vi "Add Caption and image.vi"(0 "PDF Report IN":T21(xcontrol), 2 "Caption?":bool, 5 "Paragraph Refnum":refnum<k24>, 9 "Image Ref iTexSharp":refnum<k24>, 11 "error in (no error)":errorcluster) -> (4 "PDF Report OUT":T21(xcontrol), 8 "Size (points)":cluster{"TotalHeight":sgl, "TotalWidth":sgl}, 15 "error out":errorcluster)   [LabVIEW 2012]
doc: "Version 1.0\nDeveloped by Jean-Marc Simard\nCopyright © 2010, Exaprom Inc.\nAll rights reserved.\nLicense: BSD\n\nWith iTextSharp 4.1.6 (http://itextsharp.sourceforge.net)\nunder Mozilla Public License Version 1.1\n(http://www.mozilla.org/MPL/MPL-1.1.html)"
uses:
  C:/Users/MaxCorp/Documents/GitHub/TopView/DLL/itextsharp.dll
  GitHub/TopView/DLL/itextsharp.dll
  Controls/PDF Report Xcontrol/PDF Report.xctl
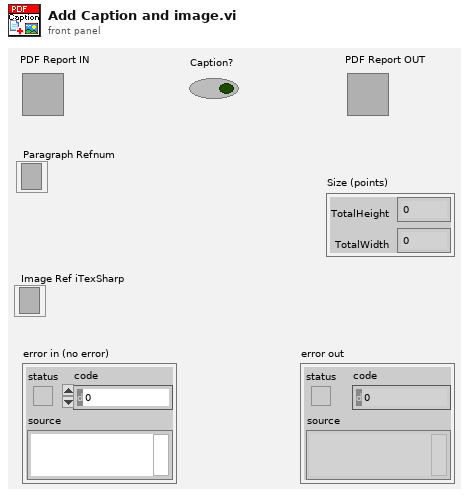
[diagram p1: front panel]
types:
  T1 = typedef "Font cluster.ctl" = cluster{"Name":string, "Size":T2, "Color":T3, "Style":cluster{"Bold":bool, "Italic":bool, "Underline":bool, "Strikeout":bool}}
  T2 = typedef "Font size.ctl" = sgl
  T3 = typedef "Font color.ctl" = u32
  T4 = typedef "Unit.ctl" = enum16{"inch", "mm"}
  T5 = typedef "Paragraphe cluster.ctl" = cluster{" Aligment":T6, "Line spacing":T7}
  T6 = typedef "Texte alignement.ctl" = enum16{"Select", "CENTER", "JUSTIFY", "LEFT", "RIGHT"}
  T7 = typedef "Line spacing.ctl" = enum16{"Select", "1.0", "1.5", "2.0"}
  T8 = typedef "Page dimensions.ctl" = cluster{"Start at page":i32, "Orientation":T9, "widht":sgl, "height":sgl, "Margin left":sgl, "Margin right":sgl, "Margin top":sgl, "Margin bottom":sgl}
  T9 = typedef "Page Orientation.ctl" = enum16{"Portrait", "Landscape"}
  T10 = typedef "Image or Table Caption.ctl" = cluster{"Caption":string, "Separator":string, "Position":enum16{"Above", "Below"}}
  T11 = typedef "Header Footer [ ].ctl" = T12[]
  T12 = typedef "Header Footer cluster.ctl" = cluster{"Start page":i32, "Type":T13, "Alignment":T14, "Vertical Alignement":T15, "Image (%)":sgl, "Page #":T16, "Text":string, "Path":string, "Font":T1, "Font refnum":refnum<k24>, "Line":cluster{"Line":T17, "Thickness (points)":sgl, "Colour":T3}}
  T13 = typedef "Header Footer Type.ctl" = enum16{"Select", "Text", "Text + hyperlink", "Page number", "Image", "Image + hyperlink"}
  T14 = typedef "Header footer horiz alignment.ctl" = enum16{"Left", "Center", "Right"}
  T15 = typedef "Cell Vertical alignment.ctl" = enum16{"TOP", "MIDDLE", "BOTTOM"}
  T16 = typedef "Page number.ctl" = cluster{"Text 1":string, "Text 2":string, "Text 3":string}
  T17 = typedef "Header Footer Line.ctl" = enum16{"No line", "Horizontal line"}
  T18 = typedef "Watermark cluster2.ctl" = cluster{"Show? (F)":bool, "Type":enum16{"Image", "Text"}, "Opacity (%)":sgl, "Rotate(°)":sgl, "Position":cluster{"Position":T19, "X":sgl, "Y":sgl}, "Image path":path, "Scaled(%)":sgl, "Image refnum":refnum<k24>, "Text":string, "Font":cluster{"Name":string, "Size":T2, "Color":T3}, "Font refnum":refnum<k24>, "Alignment":T14, "Automatic":bool}
  T19 = typedef "Watermark Position.ctl" = enum16{"Absolute", "Center (page)", "Center (text section)"}
  T20 = typedef "System Fonts.ctl" = cluster{"Font name [ ]":string[], "Font and file names [ ]":cluster{"Font name":string, "File name":string}[]}
  T21 = cluster{"Document":refnum<k24>, "Writer":refnum<k24>, "Default Font":refnum<k24>, "Default Font cluster":T1, "Path":path, "Unit (default = mm)":T4, "Paragraphe cluster":T5, "Pages dimensions [ ]":T8[], "Captions":cluster{"Image":T10, "Image counter":u16, "Table":T10, "Table counter":u16, "Font":T1}, "Header":T11, "Footer":T11, "Watermark ":T18, "Actual VI name":string, "System Fonts":T20}
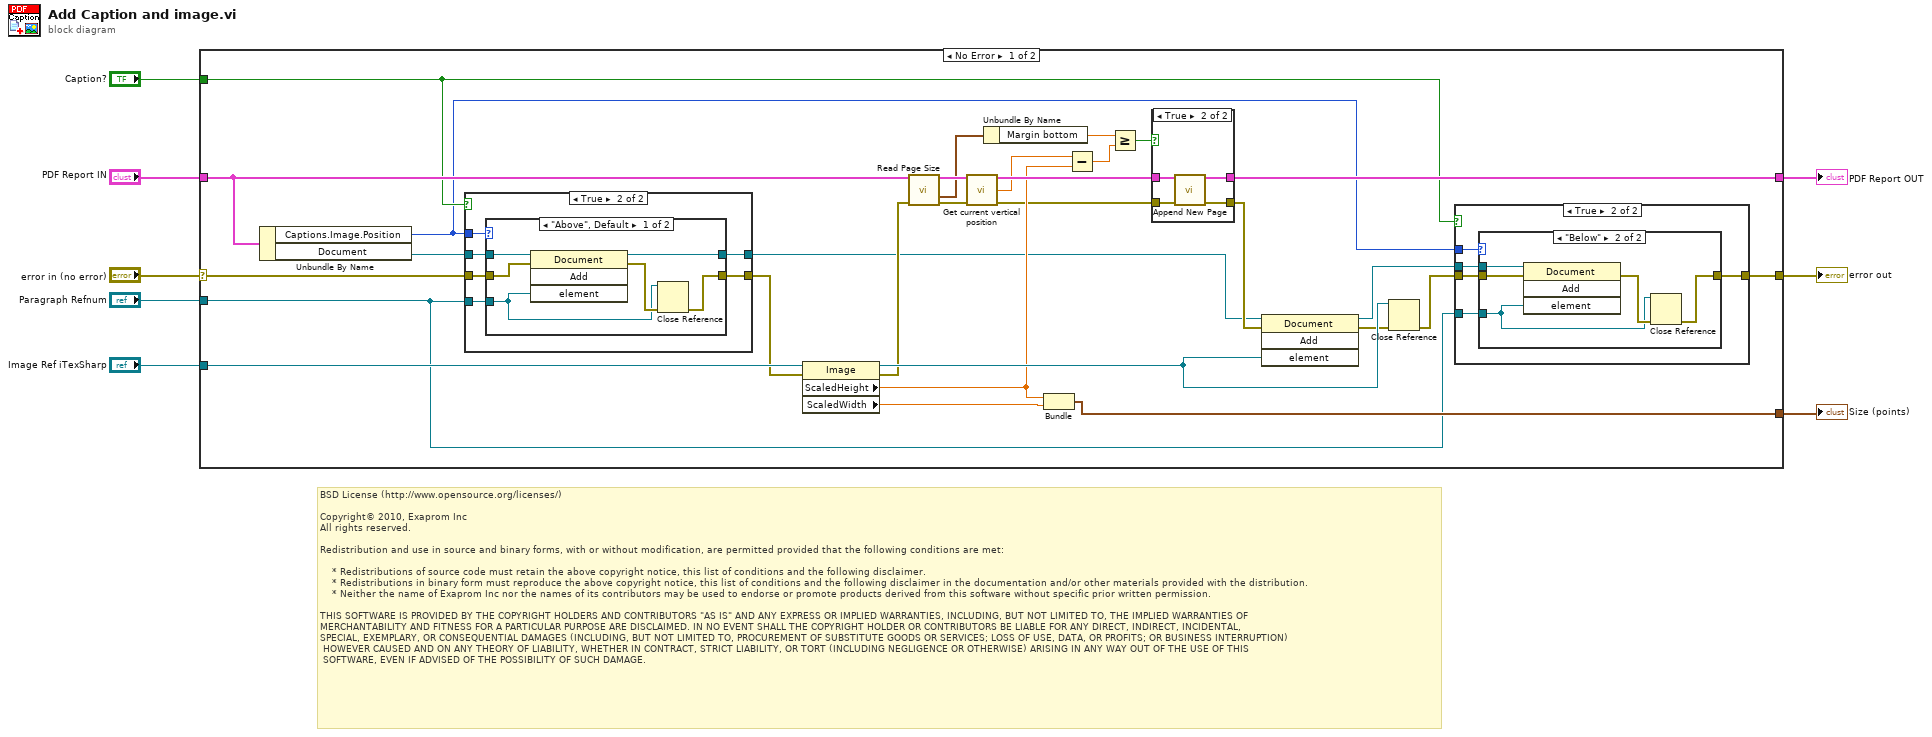
[diagram p0: block diagram]
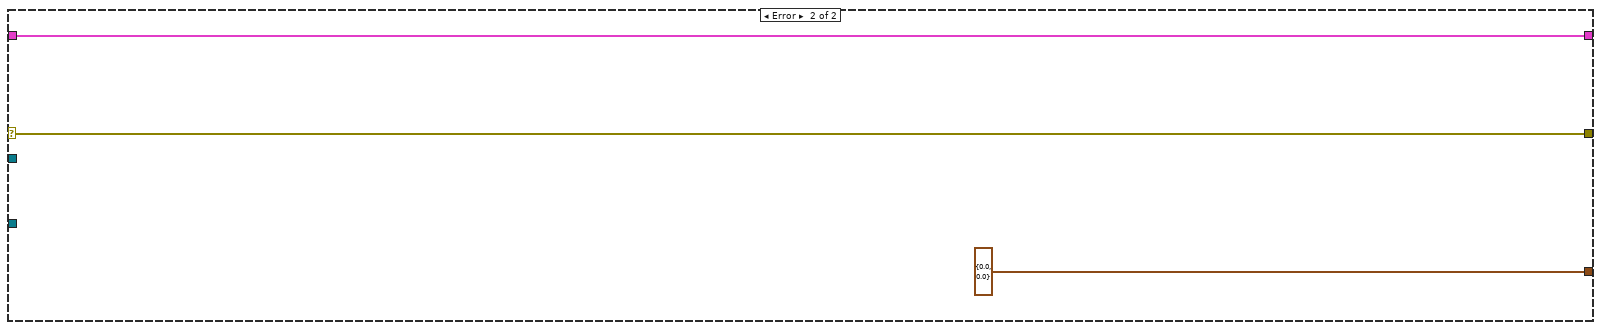
[diagram p7: hidden frame]
diagram:
  # "BSD License (http://www.opensource.org/licenses/)\n\nCopyright© 2010, Exaprom Inc\nAll rights reserved.\n\nRedistribution and use in source and binary forms, with or without modification, are permitted provided that the following conditions are met:\n\n    * Redistributions of source code must retain the above copyright notice, this list of conditions and the following disclaimer.\n    * Redistributions in binary form must reproduce the above copyright notice, this list of conditions and the following disclaimer in the documentation and/or other materials provided with the distribution.\n    * Neither the name of Exaprom Inc nor the names of its contributors may be used to endorse or promote products derived from this software without specific prior written permission.\n\nTHIS SOFTWARE IS PROVIDED BY THE COPYRIGHT HOLDERS AND CONTRIBUTORS \"AS IS\" AND ANY EXPRESS OR IMPLIED WARRANTIES, INCLUDING, BUT NOT LIMITED TO, THE IMPLIED WARRANTIES OF \nMERCHANTABILITY AND FITNESS FOR A PARTICULAR PURPOSE ARE DISCLAIMED. IN NO EVENT SHALL THE COPYRIGHT HOLDER OR CONTRIBUTORS BE LIABLE FOR ANY DIRECT, INDIRECT, INCIDENTAL,\nSPECIAL, EXEMPLARY, OR CONSEQUENTIAL DAMAGES (INCLUDING, BUT NOT LIMITED TO, PROCUREMENT OF SUBSTITUTE GOODS OR SERVICES; LOSS OF USE, DATA, OR PROFITS; OR BUSINESS INTERRUPTION)\n HOWEVER CAUSED AND ON ANY THEORY OF LIABILITY, WHETHER IN CONTRACT, STRICT LIABILITY, OR TORT (INCLUDING NEGLIGENCE OR OTHERWISE) ARISING IN ANY WAY OUT OF THE USE OF THIS\n SOFTWARE, EVEN IF ADVISED OF THE POSSIBILITY OF SUCH DAMAGE."
  n1 = case shown="No Error" "error in (no error)" {
    selector: "error in (no error)" -> [w31 w74]
    tunnel: "PDF Report IN" -> [w34 w73]
    tunnel: [w37 w73] -> w7
    tunnel: [w35 w74] -> w6
    tunnel: [w36 cluster{"ScaledHeight":sgl, "ScaledWidth":sgl} {"ScaledHeight"=0.0, "ScaledWidth"=0.0}] -> w3
    tunnel: "Image Ref iTexSharp" -> [w32 _]
    tunnel: "Caption?" -> [w29 _]
    tunnel: "Paragraph Refnum" -> [w30 _]
    frame No Error {
      n2 = Unbundle By Name(w34) -> ("Captions.Image.Position"=w9:enum16{"Above", "Below"}, "Document"=w33:refnum<k24>)
      n3 = case shown="True" w29 {
        tunnel: w31 -> [w50 w57]
        tunnel: w33 -> [w51 w56]
        tunnel: [w50 w55] -> w13
        tunnel: [w51 w54] -> w12
        tunnel: w9 -> [_ w53]
        tunnel: w30 -> [_ w52]
        frame False {
        }
        frame True {
          n4 = case shown="\"Above\", Default" w53 {
            tunnel: w52 -> [w62 _]
            tunnel: w57 -> [w61 w64]
            tunnel: [w60 w64] -> w55
            tunnel: w56 -> [w59 w65]
            tunnel: [w58 w65] -> w54
            frame "Above", Default {
              n5 = invoke class="Document" method="Add"(reference=w59, error in=w61, "element"=w62) -> (reference out=w58:refnum<k24>, error out=w63:errorcluster)  [unwired: 1 in, 2 out]
              n6 = Close Reference(reference=w62, error in (no error)=w63) -> (error out=w60:errorcluster)
            }
            frame "Below" {
            }
          }
        }
      }
      n7 = property class="Image"(reference=w32, error in=w13) -> (reference out=w28:refnum<k24>, error out=w19:errorcluster, "ScaledHeight"=w20:sgl, "ScaledWidth"=w27:sgl)
      n8 = call "Read Page Size.vi"("PDF Report"=w34, "error in (no error)"=w19) -> ("PDF Report duplicate"=w25:T21, "Page (points)"=w23:T8, "error out"=w24:errorcluster)  [unwired: 11 out]
      n9 = call "Get current vertical position.vi"("PDF Report In"=w25, "error in (no error)"=w24) -> ("PDF Report duplicate"=w26:T21, "GetVerticalPosition (points)"=w21:sgl, "error out"=w16:errorcluster)  [unwired: 1 in, 10 out]
      n10 = Unbundle By Name(w23) -> ("Margin bottom"=w22:sgl)
      n11 = Bundle("ScaledHeight"=w20, "ScaledWidth"=w27) -> (w36:cluster{"ScaledHeight":sgl, "ScaledWidth":sgl})  [unwired: 1 out]
      n12 = Subtract(x=w21, y=w20) -> (x-y=w18:sgl)
      n13 = Greater Or Equal?(x=w22, y=w18) -> (x >= y?=w17:bool)
      n14 = case shown="True" w17 {
        tunnel: w26 -> [w67 w71]
        tunnel: [w67 w70] -> w37
        tunnel: w16 -> [w66 w69]
        tunnel: [w66 w68] -> w15
        frame False {
        }
        frame True {
          n15 = call "Append New Page.vi"("PDF Report"=w71, "error in (no error)"=w69) -> ("PDF Report duplicate"=w70:T21, "error OUT"=w68:errorcluster)  [unwired: 12 out]
        }
      }
      n16 = invoke class="Document" method="Add"(reference=w12, error in=w15, "element"=w28) -> (reference out=w11:refnum<k24>, error out=w14:errorcluster)  [unwired: 1 in, 2 out]
      n17 = Close Reference(reference=w28, error in (no error)=w14) -> (error out=w10:errorcluster)
      n18 = case shown="True" w29 {
        tunnel: w9 -> [_ w43]
        tunnel: w11 -> [_ w42]
        tunnel: w30 -> [_ w41]
        tunnel: w10 -> [w38 w40]
        tunnel: [w38 w39] -> w35
        frame False {
        }
        frame True {
          n19 = case shown="\"Below\"" w43 {
            tunnel: w41 -> [_ w48]
            tunnel: w40 -> [w44 w47]
            tunnel: [w44 w46] -> w39
            tunnel: w42 -> [_ w45]
            frame "Above", Default {
            }
            frame "Below" {
              n20 = invoke class="Document" method="Add"(reference=w45, error in=w47, "element"=w48) -> (error out=w49:errorcluster)  [unwired: 1 in, 3 out]
              n21 = Close Reference(reference=w48, error in (no error)=w49) -> (error out=w46:errorcluster)
            }
          }
        }
      }
    }
    frame Error {
    }
  }
  "PDF Report OUT" <- w7
  "error out" <- w6
  "Size (points)" <- w3
